vi "New JSON (String[]).vi"(8 "error in (no error)":errorcluster, 10 "String Array":string[](array[string])) -> (0 "error out":errorcluster, 3 "JSON Value out":refnum<class "JSON Value.lvclass">)   [LabVIEW 2016, in "JSON Value.lvclass"]
doc: "Creates a new JSON Array initialized with JSON Boolean objects of the values specified by String Array"
uses:
  JSON Value.lvclass
  New JSON (String).vi
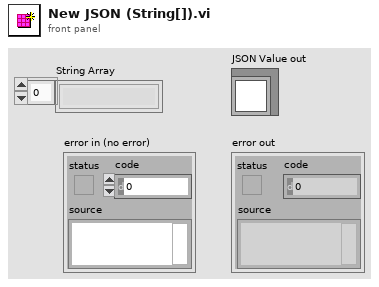
[diagram p1: front panel]
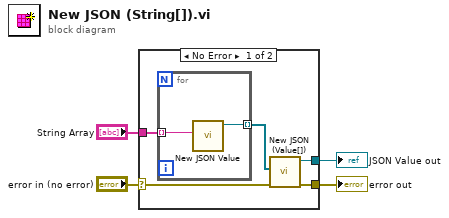
[diagram p0: block diagram]
diagram:
  n1 = case shown="No Error" "error in (no error)" {
    selector: "error in (no error)" -> [w6 w12]
    tunnel: [w5 w12] -> w3
    tunnel: [w8 _] -> w2
    tunnel: "String Array" -> [w9 _]
    frame No Error {
      n2 = for {
        tunnel: w9 -> [w11] mode=indexing
        tunnel: [w10] -> w7 mode=indexing
        n3 = call-poly "New JSON Value.vi"("value"=w11) -> ("JSON Value out"=w10:refnum<class "JSON Value.lvclass">)  [unwired: 9 in, 1 out]
      }
      n4 = call "New JSON (Value[]).vi"("error in (no error)"=w6, "JSON Datatypes"=w7) -> ("error out"=w5:errorcluster, "JSON Value out"=w8:refnum<class "JSON Value.lvclass">)  [unwired: 8 in]
    }
    frame Error {
    }
  }
  "error out" <- w3
  "JSON Value out" <- w2
